vi "Get Start and End Indices of Fast Tree.vi"(11 "Node":T1) -> (1 "Index":i32, 3 "Length":i32)   [LabVIEW 2019, in "ParseGDSII.lvclass"]
uses:
  ParseGDSII.lvclass
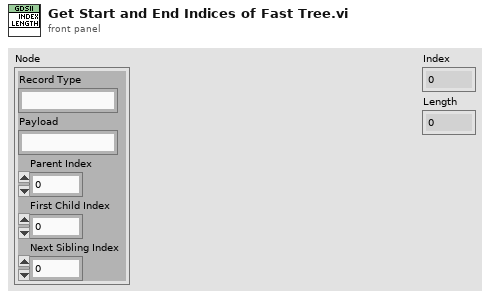
[diagram p1: front panel]
types:
  T1 = cluster{"Record Type":string, "Payload":string, "Parent Index":i32, "First Child Index":i32, "Next Sibling Index":i32}
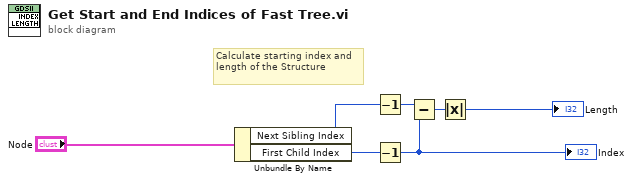
[diagram p0: block diagram]
diagram:
  # "Calculate starting index and length of the Structure"
  n1 = Unbundle By Name("Node") -> ("Next Sibling Index"=w7:i32, "First Child Index"=w6:i32)
  n2 = Decrement(x=w7) -> (x-1=w5:i32)
  n3 = Decrement(x=w6) -> (x-1=w3:i32)
  "Index" <- w3
  n4 = Subtract(x=w5, y=w3) -> (x-y=w4:i32)
  n5 = Absolute Value(x=w4) -> (abs(x)=→"Length":i32)
